vi "NanonisPos.vi"(9 "z":dbl, 10 "x":dbl, 11 "PIN":dbl) -> (3 "POUT":dbl)   [LabVIEW 2017]
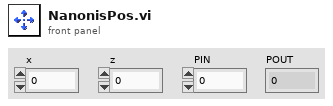
[diagram p1: front panel]
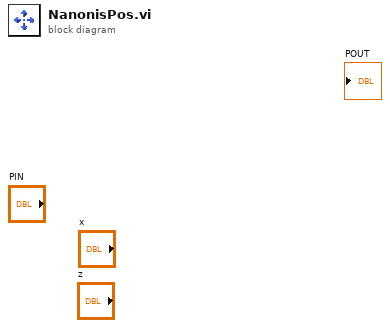
[diagram p0: block diagram]
diagram:
